vi "niRFUtil FTW Generate No FIR Filter.vi"(1 "Minimum Selectivity (dB)":dbl=70.0 format="%.2f", 2 "Sampling Rate (Hz)":dbl=2160000.0 format="%^.3e", 3 "Bandwidth (Hz)":dbl=300000.0 format="%^.3e") -> (0 "Filter":T1={"x0"=-2.777777777777778e-06, "dx"=4.6296296296296297e-07, "y"=[]} {"y" min=0 max=127 format="%.2f"; "dx" format="%^.2e"; "x0" format="%^.2e"})   [LabVIEW 2015, in "niRFUtil.lvlib"]
doc: "(c) Copyright 2006, National Instruments, Inc. This VI may not be duplicated, sold, or distributed without written consent from National Instruments."
uses:
  niRFUtil.lvlib
  Includes/niRFUtil INC Real Waveform.ctl
  Includes/niRFUtil INC Real Array.ctl
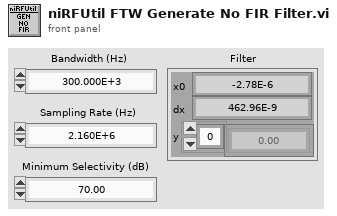
[diagram p1: front panel]
types:
  T1 = typedef "niRFUtil.lvlib/niRFUtil INC Real Waveform.ctl" = cluster{"x0":dbl, "dx":dbl, "y":T2}
  T2 = typedef "niRFUtil.lvlib/niRFUtil INC Real Array.ctl" = sgl[]
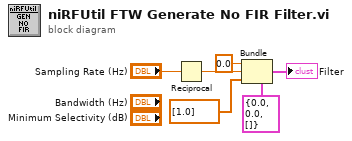
[diagram p0: block diagram]
diagram:
  n1 = Reciprocal(x="Sampling Rate (Hz)") -> (1/x=w3:dbl)
  n2 = Bundle(cluster=T1 {"x0"=0.0, "dx"=0.0, "y"=[]} ("Filter"), "x0"=0.0, "dx"=w3, "y"=T2 [1.0]) -> (→"Filter":T1)
